vi "decoder.vi"(1 "rsp package":string, 2 "byte count":i32) -> (0 "output cluster":T1)   [LabVIEW 2020]
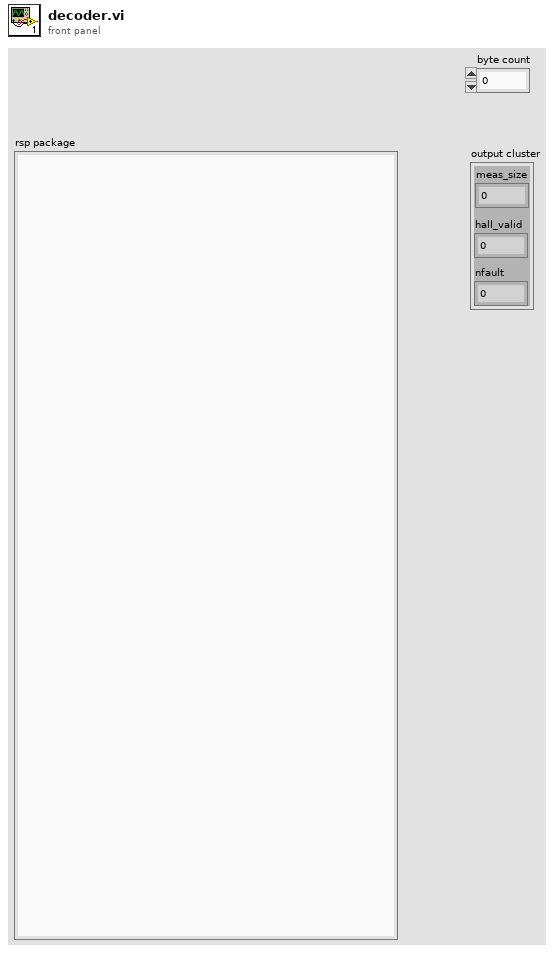
[diagram p1: front panel]
types:
  T1 = cluster{"meas_size":dbl, "hall_valid":u8, "nfault":u8}
  T2 = cluster{dbl[], dbl[], dbl[], dbl[], dbl, dbl, dbl}
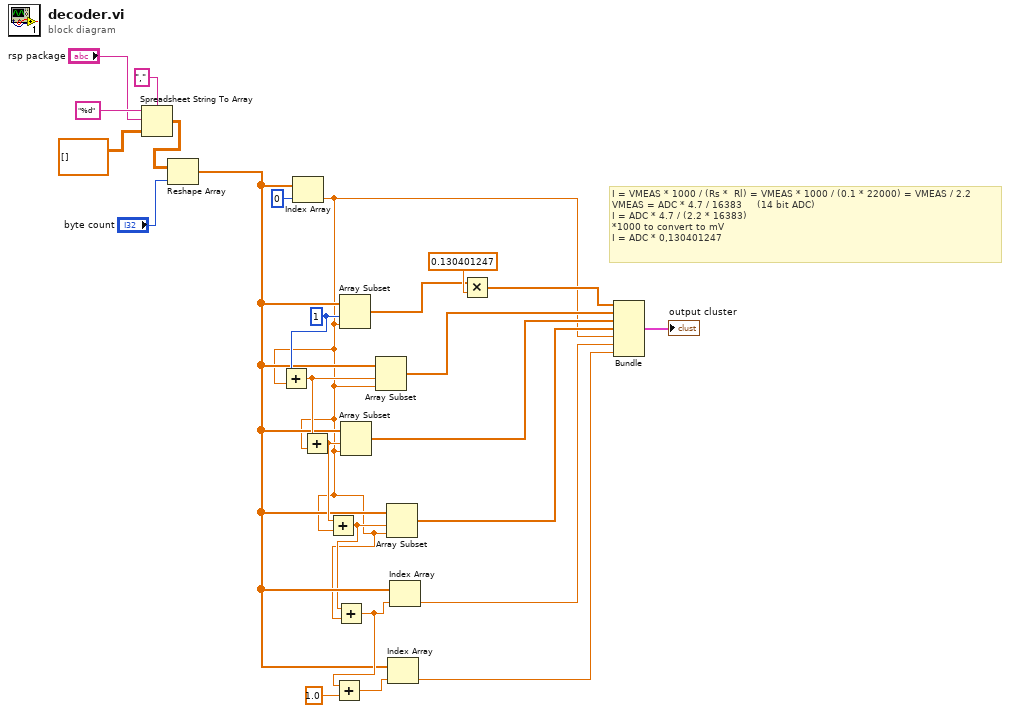
[diagram p0: block diagram]
diagram:
  w13 = 1 ("index")
  # "I = VMEAS * 1000 / (Rs *  Rl) = VMEAS * 1000 / (0.1 * 22000) = VMEAS / 2.2 \nVMEAS = ADC * 4.7 / 16383     (14 bit ADC)\nI = ADC * 4.7 / (2.2 * 16383)\n*1000 to convert to mV\nI = ADC * 0,130401247"
  n1 = Spreadsheet String To Array(delimiter (Tab)=",", format string="%d", spreadsheet string="rsp package", array type (2D Dbl)=dbl[][] []) -> (array=w22:dbl[][])
  n2 = Reshape Array(w22, "byte count") -> (w4:dbl[])
  n3 = Index Array "Index Array"(array=w4, index=0) -> (element=w1:dbl)
  n4 = Add(x=w13, y=w1) -> (x+y=w12:dbl)
  n5 = Add(x=w12, y=w1) -> (x+y=w5:dbl)
  n6 = Add(x=w5, y=w1) -> (x+y=w2:dbl)
  n7 = Add(x=w2, y=w1) -> (x+y=w8:dbl)
  n8 = Add(x=w8, y=1.0) -> (x+y=w10:dbl)
  n9 = Array Subset "Array Subset"(array=w4, index=w13, length=w1) -> (w20:dbl[])
  n10 = Array Subset(array=w4, index=w5, length=w1) -> (w16:dbl[])
  n11 = Array Subset(array=w4, index=w12, length=w1) -> (w17:dbl[])
  n12 = Array Subset(array=w4, index=w2, length=w1) -> (w3:dbl[])
  n13 = Index Array(array=w4, index=w10) -> (element=w7:dbl)
  n14 = Index Array(array=w4, index=w8) -> (element=w6:dbl)
  n15 = Multiply(x=w20, y=0.130401247) -> (x*y=w18:dbl[])
  n16 = Bundle(w18, w17, w16, w3, w1, w6, w7) -> (→"output cluster":T2)  [unwired: 1 in]
